vi "1D Parabolic Max.vi"(9 "Y":dbl[](array[numeric]), 10 "Xt":dbl, 11 "X":dbl[](array[numeric])) -> (0 "Found max":bool, 1 "Ymax":dbl, 3 "Xmax":dbl, 4 "Finer Best Polynomial Fit":dbl[](array[numeric]), 5 "Best Polynomial Fit":dbl[](array[numeric]), 6 "Y(Xt) < Ymin":bool, 7 "Y(Xt) > Ymax":bool, 8 "Finer X":dbl[](array[numeric]))   [LabVIEW 2018]
uses:
  <vilib>/Analysis/NI_AALPro.lvlib
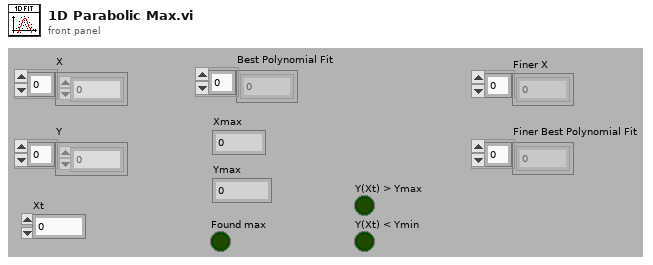
[diagram p1: front panel]
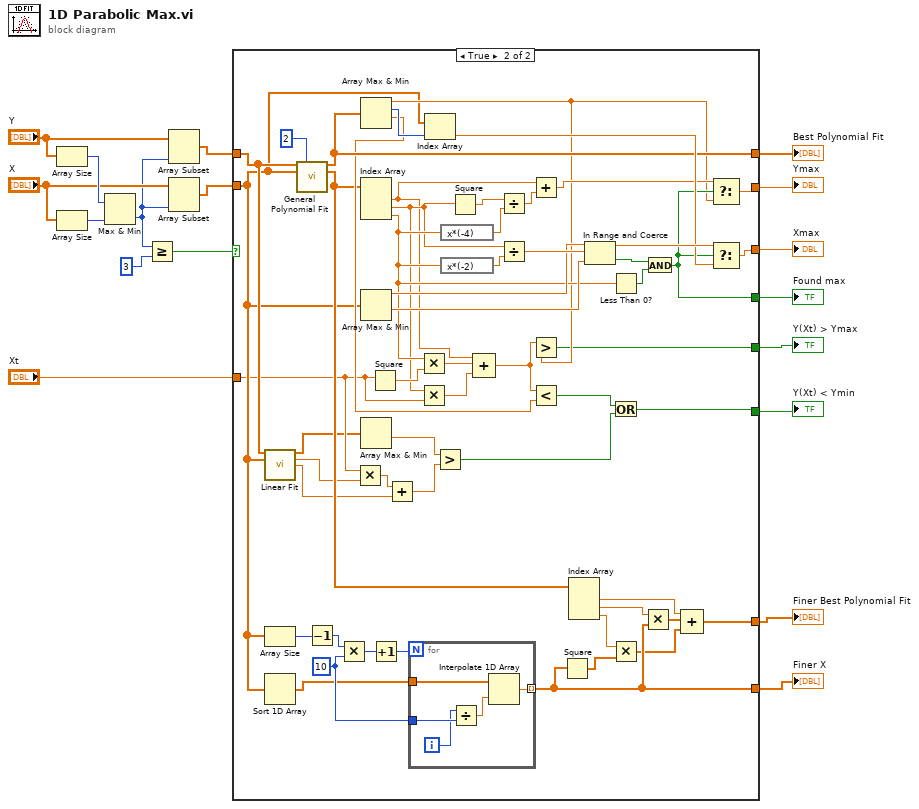
[diagram p0: block diagram]
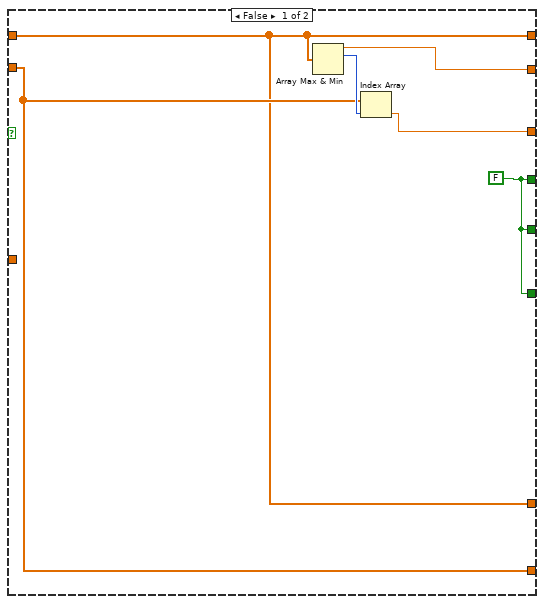
[diagram p2: hidden frame]
diagram:
  n1 = Array Size(array="Y") -> (size(s)=w12:i32)
  n2 = Array Size(array="X") -> (size(s)=w11:i32)
  n3 = Max & Min(x=w12, y=w11) -> (min(x,y)=w6:i32)  [unwired: 1 out]
  n4 = Greater Or Equal?(x=w6, y=3) -> (x >= y?=w13:bool)
  n5 = Array Subset(array="Y", length=w6) -> (w9:dbl[])  [unwired: 1 in]
  n6 = Array Subset(array="X", length=w6) -> (w8:dbl[])  [unwired: 1 in]
  n7 = case shown="True" w13 {
    tunnel: w9 -> [w19 w36]
    tunnel: [w24 w63] -> w18
    tunnel: [w22 w71] -> w17
    tunnel: [w19 w65] -> w16
    tunnel: w8 -> [w20 w35]
    tunnel: [w21 w62] -> w15
    tunnel: [w21 w52] -> w5
    tunnel: [w21 w25] -> w4
    tunnel: "Xt" -> [_ w33]
    tunnel: [w20 w43] -> w2
    tunnel: [w19 w38] -> w1
    frame False {
      w21 = FALSE
      n8 = Array Max & Min(array=w19) -> (max value=w24:dbl, max index (indices)=w23:i32)  [unwired: 2 out]
      n9 = Index Array(array=w20, index=w23) -> (element=w22:dbl)
    }
    frame True {
      w47 = 10 ("y")
      n10 = call <vilib>:"Linear Fit.vi"("Y"=w36, "X"=w35) -> ("Best Linear Fit"=w30:dbl[], "slope"=w34:dbl, "intercept"=w31:dbl)  [unwired: 9 in, 2 out]
      n11 = Array Size(array=w35) -> (size(s)=w49:i32)
      n12 = Sort 1D Array(array=w35) -> (sorted array=w37:dbl[])
      n13 = call <vilib>:"General Polynomial Fit.vi"("Y"=w36, "polynomial order"=2, "X"=w35) -> ("Best Polynomial Fit"=w65:dbl[], "Polynomial Coefficients"=w44:dbl[])  [unwired: 9 in, 2 out]
      n14 = Decrement(x=w49) -> (x-1=w51:i32)
      n15 = Multiply(x=w51, y=w47) -> (x*y=w50:i32)
      n16 = Multiply(x=w33, y=w34) -> (x*y=w32:dbl)
      n17 = Array Max & Min(array=w65) -> (max value=w55:dbl, max index (indices)=w67:i32, min value=w53:dbl)  [unwired: 1 out]
      n18 = Index Array(array=w44) -> (element #1=w56:dbl, element #2=w59:dbl, element #3=w60:dbl)  [unwired: 3 in]
      n19 = Array Max & Min(array=w35) -> (max value=w69:dbl, min value=w68:dbl)  [unwired: 2 out]
      n20 = Array Max & Min(array=w30) -> (min value=w29:dbl)  [unwired: 3 out]
      n21 = Square(x=w33) -> (x^2=w61:dbl)
      n22 = Increment(x=w50) -> (x+1=w48:i32)
      n23 = Add(x=w32, y=w31) -> (x+y=w28:dbl)
      n24 = for {
        N: w48 -> [_]
        tunnel: w37 -> [w84]
        tunnel: w47 -> [w82]
        tunnel: [w80] -> w43 mode=indexing
        i -> [w81]
        n25 = Divide(x=w81, y=w82) -> (x/y=w83:dbl)
        n26 = Interpolate 1D Array(1:w83, 2:w84) -> (0:w80:dbl)
      }
      n27 = Multiply(x=w60, y=w61) -> (x*y=w58:dbl)
      n28 = Multiply(x=w59, y=w33) -> (x*y=w57:dbl)
      n29 = Index Array(array=w35, index=w67) -> (element=w66:dbl)
      n30 = Greater?(x=w29, y=w28) -> (0:w26:bool)
      n31 = expression code="x*(-4)"(w60) -> (w76:dbl)
      n32 = expression code="x*(-2)"(w60) -> (w78:dbl)
      n33 = Square(x=w59) -> (x^2=w77:dbl)
      n34 = Compound Arithmetic op=ADD(w56, w58, w57) -> (w54:dbl)
      n35 = Divide(x=w77, y=w76) -> (x/y=w75:dbl)
      n36 = Divide(x=w59, y=w78) -> (x/y=w74:dbl)
      n37 = Add(x=w56, y=w75) -> (x+y=w64:dbl)
      n38 = Greater?(x=w54, y=w55) -> (0:w52:bool)
      n39 = Less?(x=w54, y=w53) -> (x < y?=w27:bool)
      n40 = Square(x=w43) -> (x^2=w46:dbl[])
      n41 = Index Array(array=w44) -> (element #1=w40:dbl, element #2=w42:dbl, element #3=w45:dbl)  [unwired: 3 in]
      n42 = In Range and Coerce(upper limit=w69, x=w74, lower limit=w68) -> (coerced(x)=w72:dbl, In Range?=w73:bool)
      n43 = Less Than 0?(x=w60) -> (x < 0?=w70:bool)
      n44 = Or(x=w27, y=w26) -> (x .or. y?=w25:bool)
      n45 = Multiply(x=w45, y=w46) -> (x*y=w39:dbl[])
      n46 = Multiply(x=w42, y=w43) -> (x*y=w41:dbl[])
      n47 = And(x=w73, y=w70) -> (x .and. y?=w62:bool)
      n48 = Compound Arithmetic op=ADD(w40, w41, w39) -> (w38:dbl[])
      n49 = Select(t=w64, s=w62, f=w55) -> (s? t:f=w63:dbl)
      n50 = Select(t=w72, s=w62, f=w66) -> (s? t:f=w71:dbl)
    }
  }
  "Best Polynomial Fit" <- w16
  "Xmax" <- w17
  "Ymax" <- w18
  "Found max" <- w15
  "Y(Xt) > Ymax" <- w5
  "Y(Xt) < Ymin" <- w4
  "Finer X" <- w2
  "Finer Best Polynomial Fit" <- w1
